vi "Encrypt for DSPACE.vi"(0 "ss":u32, 1 "SETTING PARAMETER:":i32, 2 "Hebe or Street":i16, 3 "velocity":u32) -> (7 "Message for dSpace":u32)   [LabVIEW 2016]
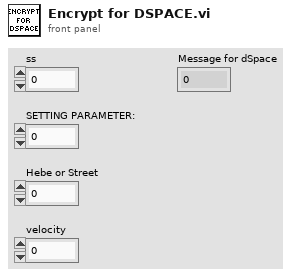
[diagram p1: front panel]
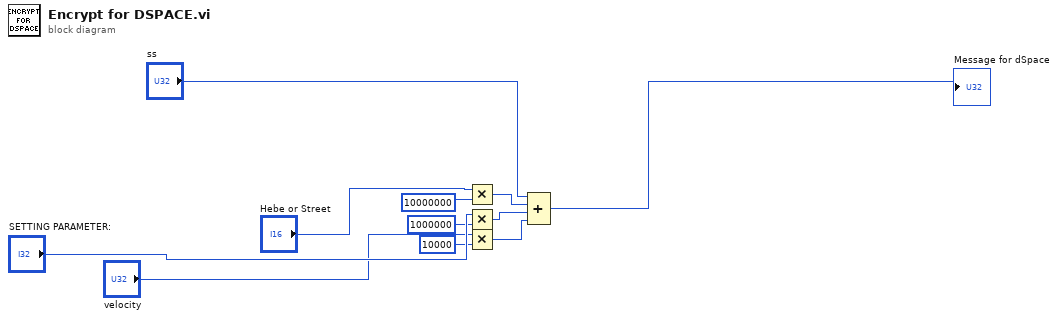
[diagram p0: block diagram]
diagram:
  n1 = Multiply(x="Hebe or Street", y=u32 10000000) -> (x*y=w6:u32)
  n2 = Multiply(x="SETTING PARAMETER:", y=u32 1000000) -> (x*y=w7:u32)
  n3 = Multiply(x="velocity", y=u32 10000) -> (x*y=w8:u32)
  n4 = Compound Arithmetic op=ADD("ss", w6, w7, w8) -> (→"Message for dSpace":u32)
